vi "Pfeiffer Vacuum OnTool General operating info.vi"(8 "error in (no error)":errorcluster, 9 "Parameter":u16(ring) items=[" Final rotation speed BkP [Hz]", " Motor current BkP [A]", " Motor voltage BkP [V]", " Motor power BkP [W]", " Operating hours BkP [h]", " Over temperature Controller (read only)", " Over temperature BkP (read only)"], 10 "Adress of unit":u16=1 min=1 max=999 step=1, 11 "COM Port Name in":refnum<visa-resource-name>="COM1") -> (0 "error out":errorcluster, 3 "response (data)":string)   [LabVIEW 2021]
doc: "This VI is an example of how to use the Pfeiffer Vacuum subVIs programmatically. This VI first initializes the instrument, takes measurements, then closes the instrument."
uses:
  <instrlib>/Pfeiffer Vacuum/Pfeiffer Vacuum.lvlib
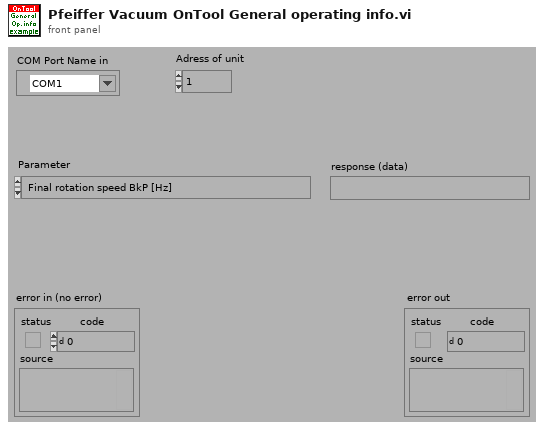
[diagram p1: front panel]
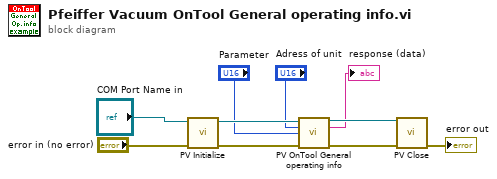
[diagram p0: block diagram]
diagram:
  n1 = call <instrlib>:"PV Initialize.vi"("error in (no error)"="error in (no error)", "VISA session in"="COM Port Name in") -> ("error out"=w8:errorcluster, "VISA session out"=w6:refnum<visa-resource-name>)  [unwired: 8 in]
  n2 = call <instrlib>:"PV OnTool General operating info.vi"("VISA session"=w6, "Adress of unit"="Adress of unit", "Parameter"="Parameter", "error in (no error)"=w8) -> ("dup VISA session"=w5:refnum<visa-resource-name>, "response (data)"=→"response (data)":string, "error out"=w7:errorcluster)  [unwired: 9 in]
  n3 = call <instrlib>:"PV Close.vi"("VISA session"=w5, "error in (no error)"=w7) -> ("error out"=→"error out":errorcluster)  [unwired: 13 in]
